vi "No Calibration.vi"(1 "Resistance, (Ohm)":dbl) -> (0 "Temperature, (K)":dbl)   [LabVIEW 2013]
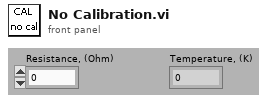
[diagram p1: front panel]
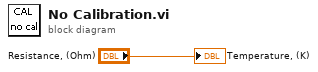
[diagram p0: block diagram]
diagram:
  "Temperature, (K)" <- "Resistance, (Ohm)"
